vi "DetectTriggerGivenTrack.vi"(8 "error in (no error)":errorcluster, 9 "CameraFrame":i32, 10 "Track":T1, 11 "StimulateReversingWorms in":refnum<class "StimulateReversingWorms.lvclass">) -> (0 "error out":errorcluster, 2 "Triggered?":bool, 3 "StimulateReversingWorms out":refnum<class "StimulateReversingWorms.lvclass">)   [LabVIEW 2019, in "StimulateReversingWorms.lvclass"]
uses:
  StimulateReversingWorms.lvclass
  WormTrackCluster.ctl
  StimulusObject.lvclass
  TrackTerminationReasonEnum.ctl
  StimulateReversingWorms.lvclass/StimulateReversingWorms.ctl
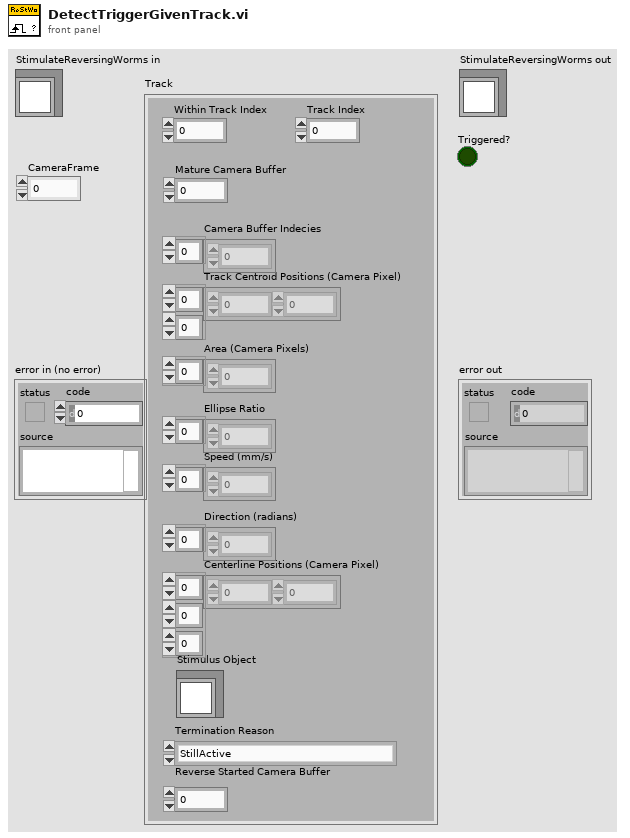
[diagram p1: front panel]
types:
  T1 = typedef "WormTrackCluster.ctl" = cluster{"Track Centroid Positions (Camera Pixel)":sgl[][], "Within Track Index":i32, "Camera Buffer Indecies":i32[], "Area (Camera Pixels)":i32[], "Speed (mm/s)":sgl[], "Direction (radians)":sgl[], "Centerline Positions (Camera Pixel)":sgl[][][], "Ellipse Ratio":sgl[], "Stimulus Object":refnum<class "StimulusObject.lvclass">, "Termination Reason":T2, "Track Index":i32, "Mature Camera Buffer":i32, "Reverse Started Camera Buffer":i32}
  T2 = typedef "TrackTerminationReasonEnum.ctl" = enum16{"StillActive", "MaxDisplacement", "NoBlobsLeft", "AreaIncrease", "AreaDecrease", "ExperimentEnded"}
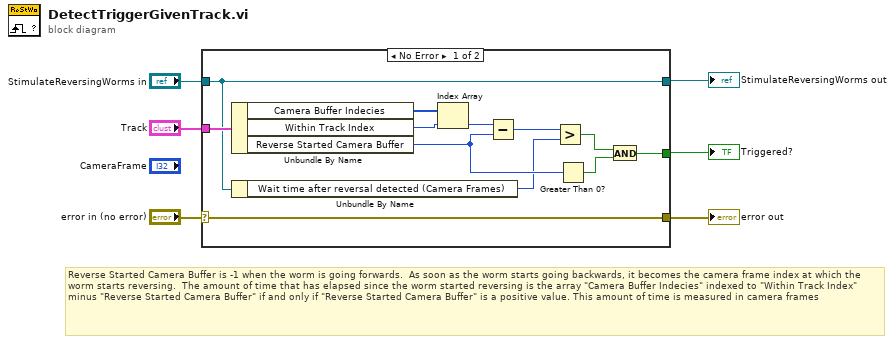
[diagram p0: block diagram]
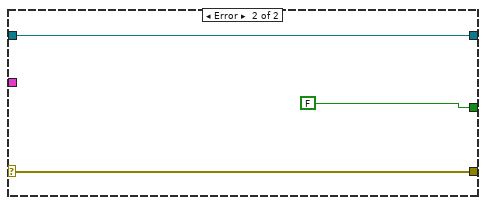
[diagram p2: hidden frame]
diagram:
  # "Reverse Started Camera Buffer is -1 when the worm is going forwards.  As soon as the worm starts going backwards, it becomes the camera frame index at which the worm starts reversing.  The amount of time that has elapsed since the worm started reversing is the array \"Camera Buffer Indecies\" indexed to \"Within Track Index\" minus \"Reverse Started Camera Buffer\" if and only if \"Reverse Started Camera Buffer\" is a positive value. This amount of time is measured in camera frames"
  n1 = case shown="No Error" "error in (no error)" {
    selector: "error in (no error)" -> [w13 w21]
    tunnel: [w13 w21] -> w3
    tunnel: "StimulateReversingWorms in" -> [w8 w20]
    tunnel: [w8 w20] -> w1
    tunnel: "Track" -> [w18 _]
    tunnel: [w9 FALSE] -> w2
    frame No Error {
      n2 = Unbundle By Name(w18) -> ("Camera Buffer Indecies"=w17:i32[], "Within Track Index"=w16:i32, "Reverse Started Camera Buffer"=w12:i32)
      n3 = Unbundle By Name(w8) -> ("Wait time after reversal detected (Camera Frames)"=w7:i32)
      n4 = Index Array(array=w17, index=w16) -> (element=w15:i32)
      n5 = Subtract(x=w15, y=w12) -> (x-y=w14:i32)
      n6 = Greater?(x=w14, y=w7) -> (0:w11:bool)
      n7 = Greater Than 0?(x=w12) -> (x > 0?=w10:bool)
      n8 = And(x=w11, y=w10) -> (x .and. y?=w9:bool)
    }
    frame Error {
    }
  }
  "error out" <- w3
  "StimulateReversingWorms out" <- w1
  "Triggered?" <- w2
